vi "Close SHVs.vi"(8 "error in (no error)":errorcluster, 11 "AMS Gas in":refnum<class "AMS Gas.lvclass">) -> (0 "error out":errorcluster, 3 "AMS Gas out":refnum<class "AMS Gas.lvclass">)   [LabVIEW 2015, in "AMS UI.lvlib" / "AMS Gas.lvclass"]
uses:
  AMS Gas.lvclass
  AMS Gas.lvclass/AMS Gas.ctl
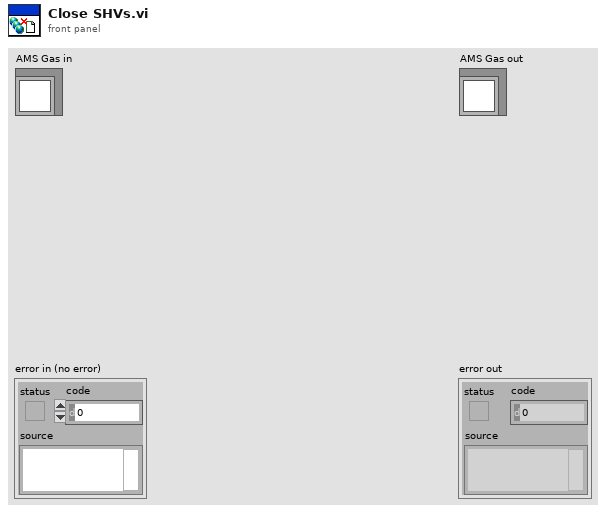
[diagram p1: front panel]
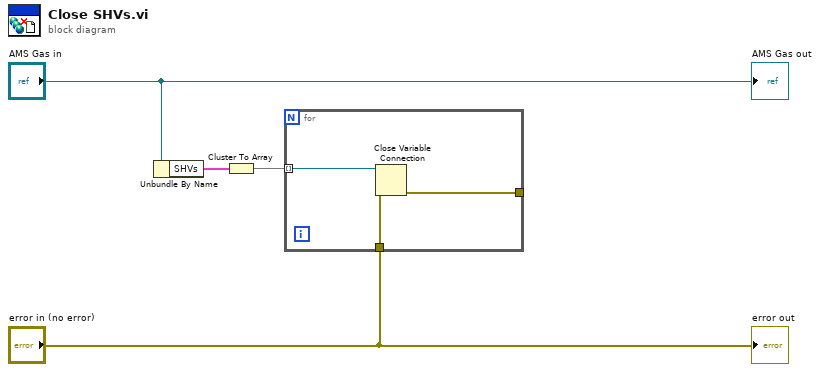
[diagram p0: block diagram]
diagram:
  n1 = Unbundle By Name("AMS Gas in") -> ("SHVs"=w4:cluster{"Sample Transfer State":refnum<k21>})
  n2 = Cluster To Array(cluster=w4) -> (array=w2:refnum<k21>[])
  n3 = for {
    tunnel: w2 -> [w7] mode=indexing
    tunnel: "error in (no error)" -> [w6]
    tunnel: [w5] -> _
    n4 = Close Variable Connection(8:w6, 11:w7) -> (0:w5:errorcluster)
  }
  "error out" <- "error in (no error)"
  "AMS Gas out" <- "AMS Gas in"
